vi "Extended Actor Template-Core_Process.vi"(0 "FTW Actor Instance Configuration":string="{\n  \"Identity\": \"ActorName\",\n  \"InboxAddress\": \"inproc://*\",\n  \"LoggerAddress\": \"\",\n  \"DebugEnableInboxLogging\": false,\n  \"DebugEnableJobLogging\": false,\n  \"LauncherAddress\": \"\",\n  \"Connections\": {\n    \"ConnectionOne\": \"inproc://connection-one\",\n    \"ConnectionTwo\": \"tcp://localhost/connection-two\"\n  },\n  \"Publishers\": {\n    \"PublisherOne\": \"inproc://publisher-one\",\n    \"PublisherTwo\": \"tcp://localhost/publisher-two\"\n  },\n  \"Subscriptions\": {\n    \"SubscriptionOne\": \"inproc://subscription-one\",\n    \"SubscriptionTwo\": \"tcp://localhost/subscription-two\"\n  },\n  \"My Data\": false,\n  \"Refresh Period\": 2\n}", 11 "ErrorIn":errorcluster) -> (15 "Error":errorcluster)   [LabVIEW 2013, in "Extended Actor Template-Core.lvclass"]
uses:
  Extended Actor Template-Core.lvclass
  source/actor/Message/Base/FTW-Message.lvclass
  Extended Actor Template-Core.lvclass/Extended Actor Template-Core.ctl
  source/actor/Instance/FTW-ActorInstance.lvclass/FTW-ActorInstance.ctl
  source/actor/JobSequencer/FTW-SEQ-Current.vi
  source/actor/Instance/FTW-ActorInstance.lvclass
  source/actor/Message/Request/FTW-Message-IncomingRequest.lvclass
  source/actor/Instance-Extended/FTW-ActorExtended.lvclass
panel:
  # "#TODO\nhide controls for a GUI"
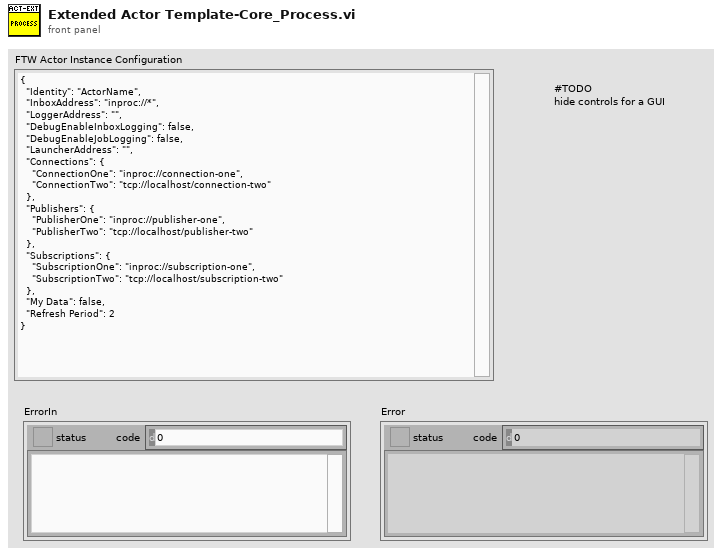
[diagram p1: front panel]
types:
  T1 = cluster{"Incoming Requests":refnum<event-registration>, "Local Messages":refnum<event-registration>, "Subscriber Registration":refnum<event-registration>}
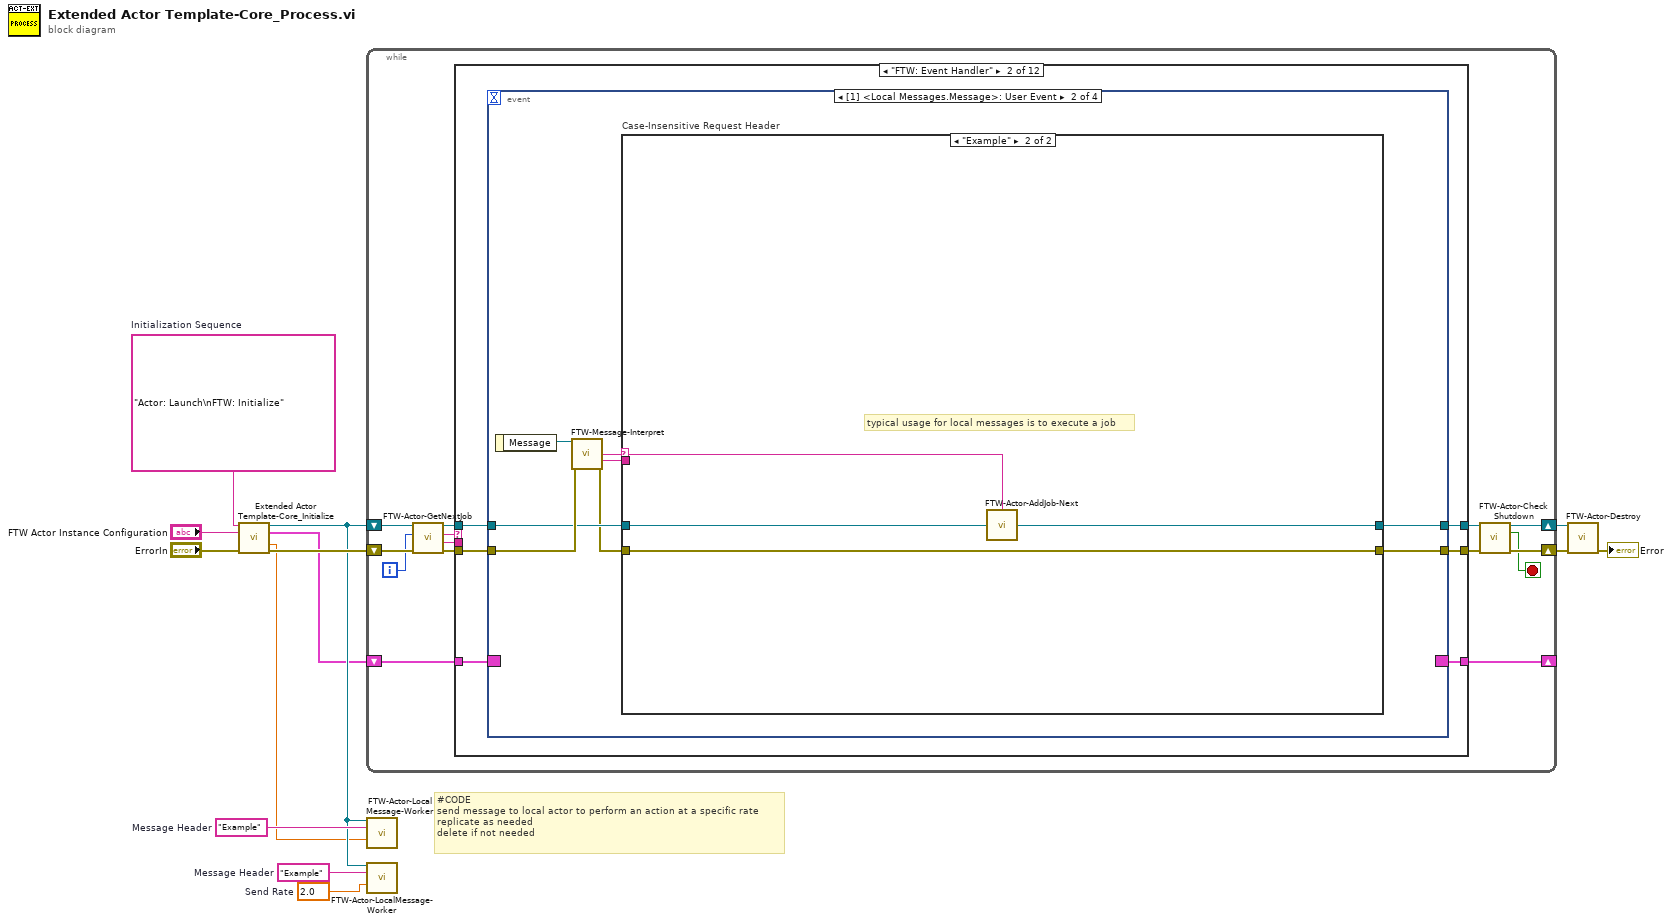
[diagram p0: block diagram]
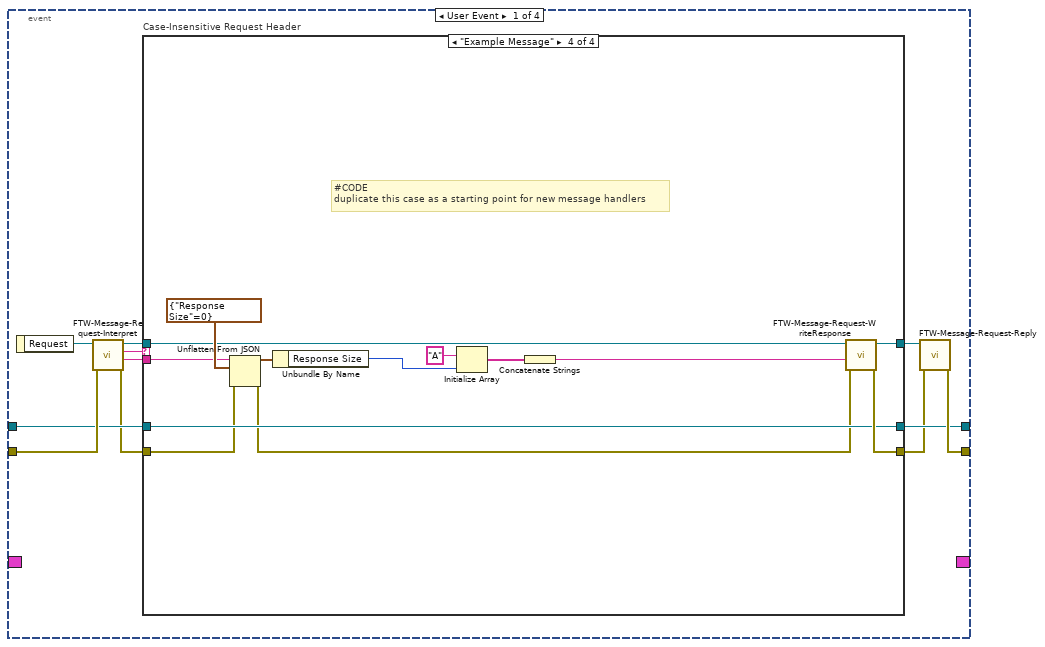
[diagram p3: hidden frame]
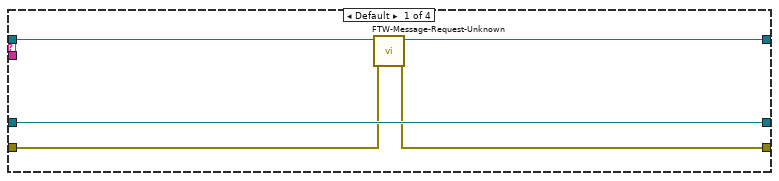
[diagram p4: hidden frame]
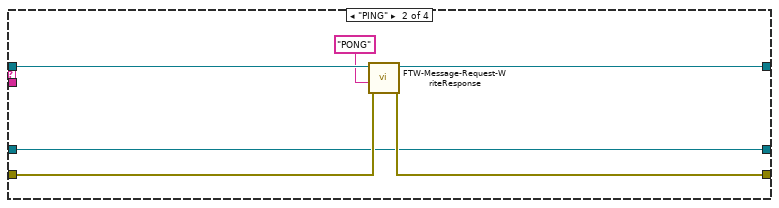
[diagram p5: hidden frame]
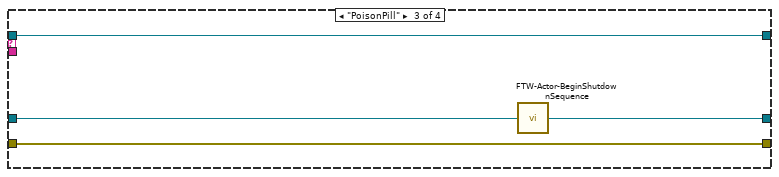
[diagram p6: hidden frame]
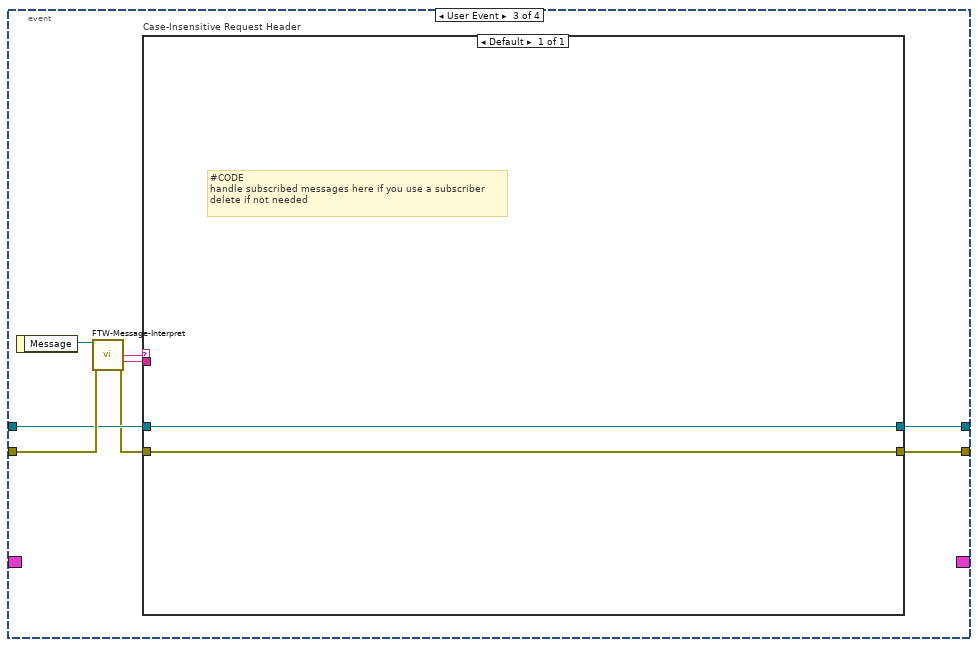
[diagram p8: hidden frame]
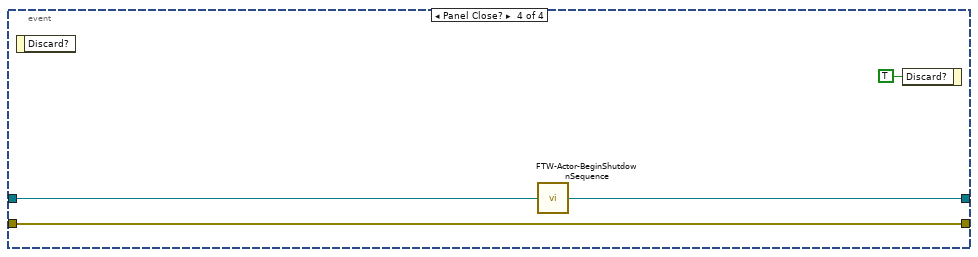
[diagram p9: hidden frame]
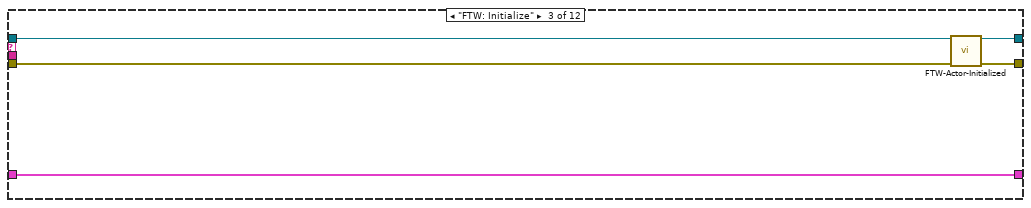
[diagram p10: hidden frame]
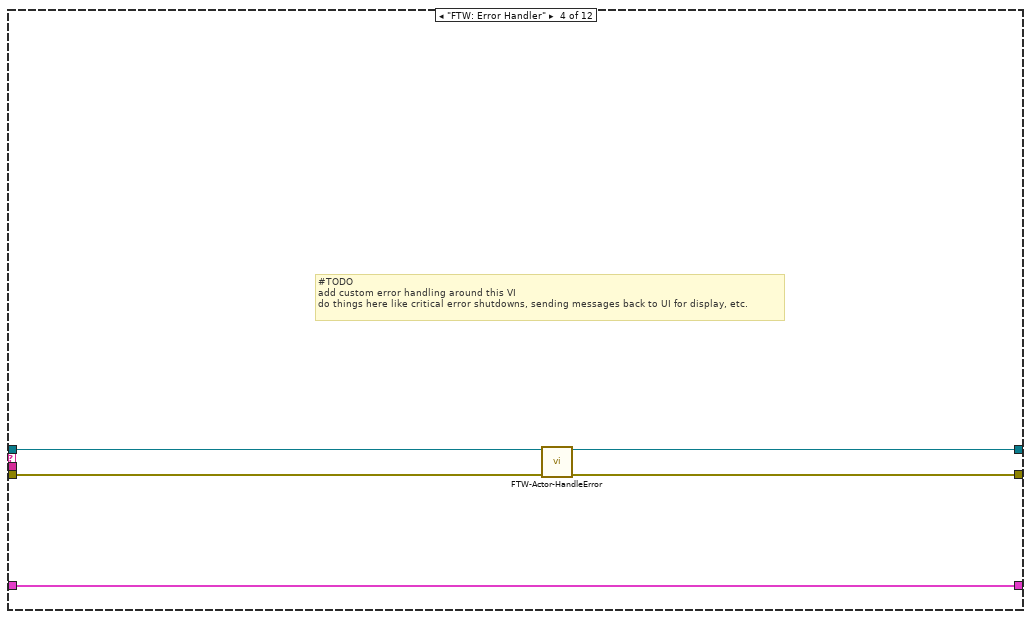
[diagram p11: hidden frame]
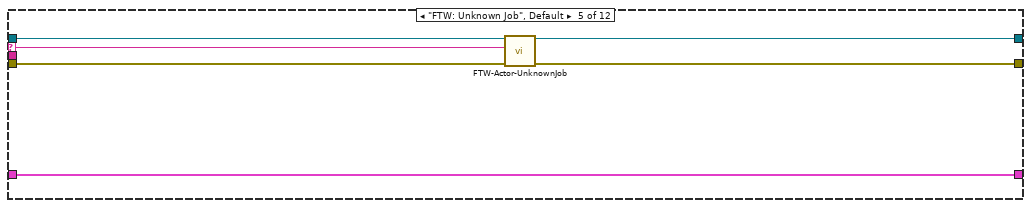
[diagram p12: hidden frame]
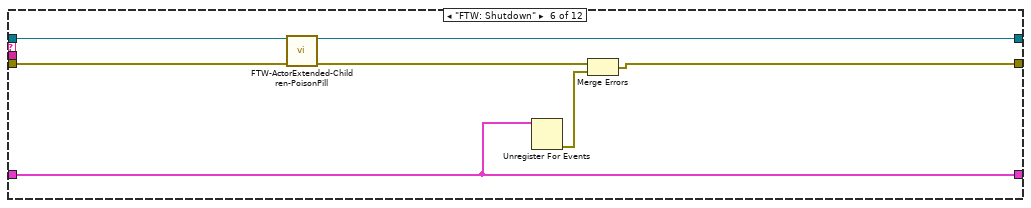
[diagram p13: hidden frame]
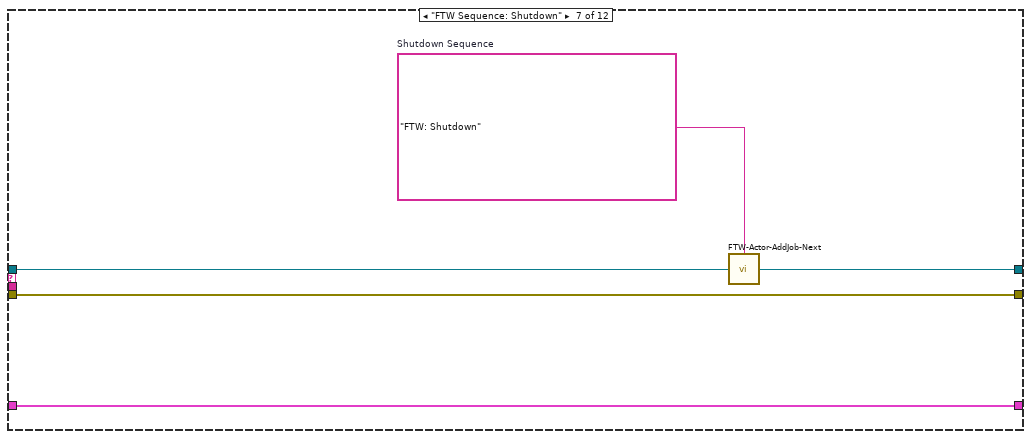
[diagram p14: hidden frame]
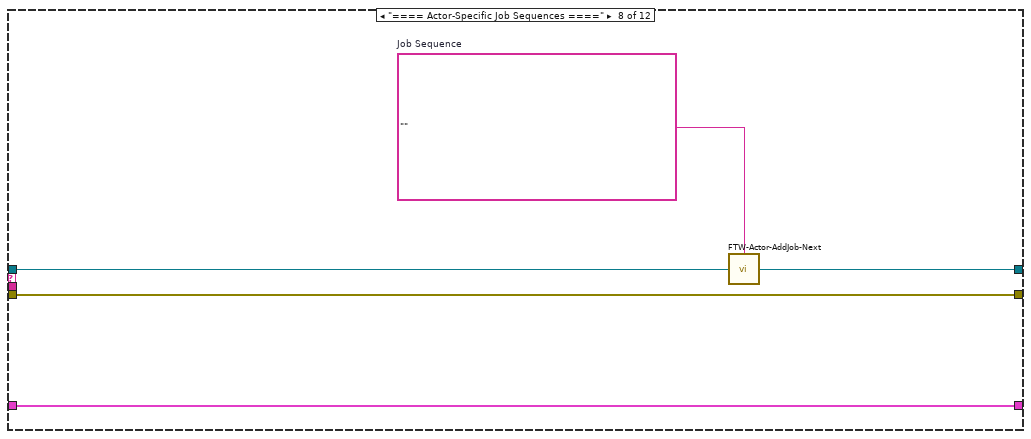
[diagram p15: hidden frame]
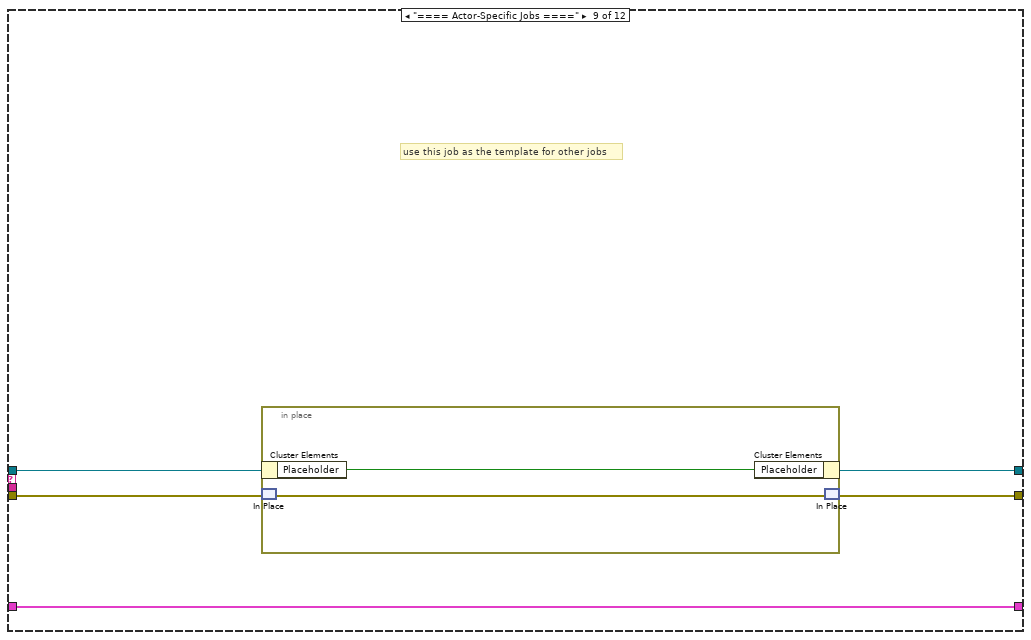
[diagram p16: hidden frame]
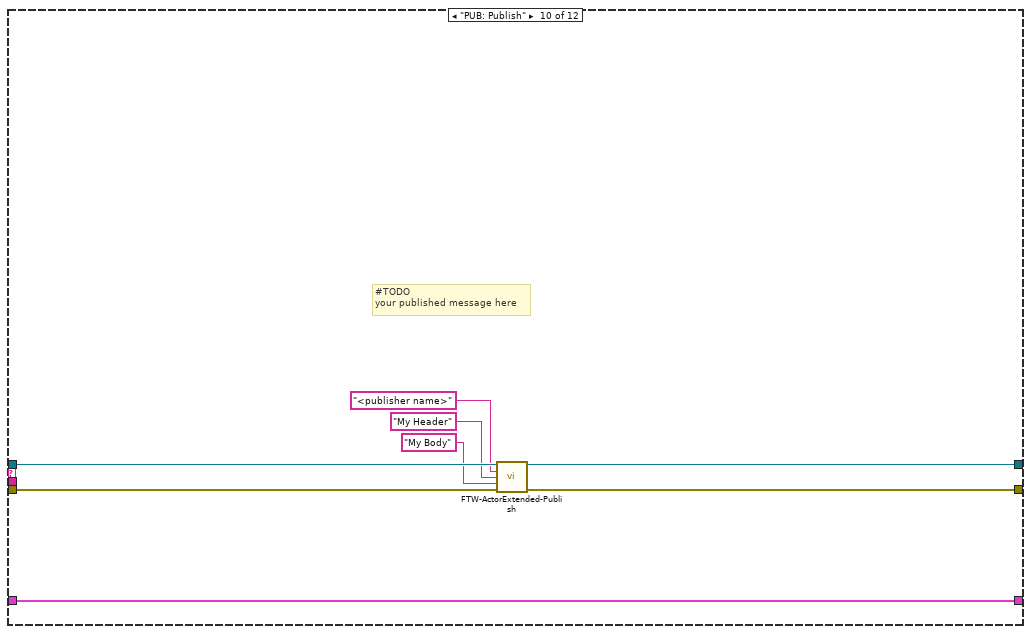
[diagram p17: hidden frame]
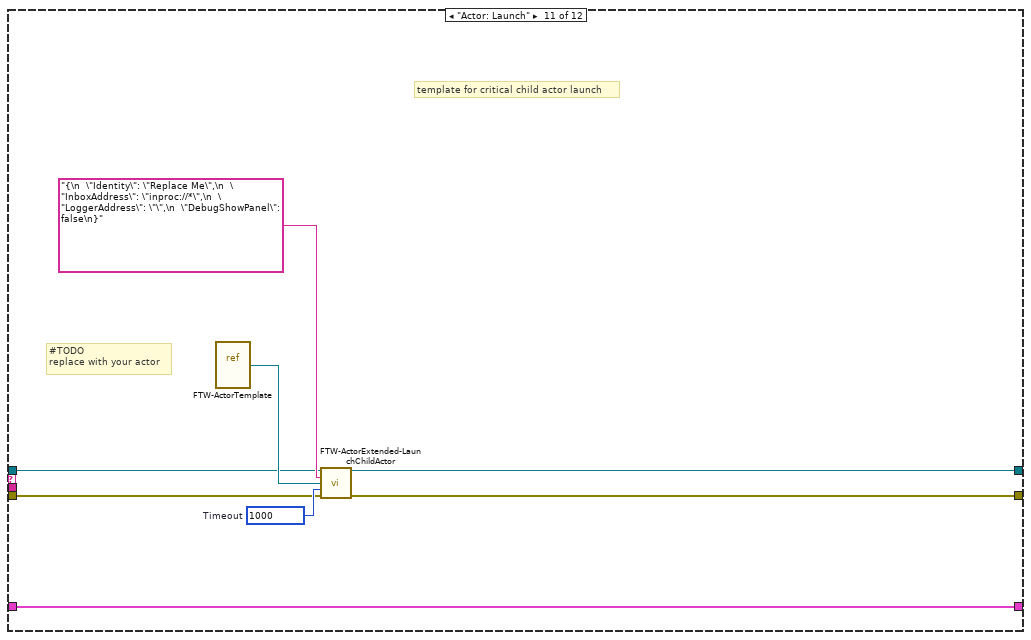
[diagram p18: hidden frame]
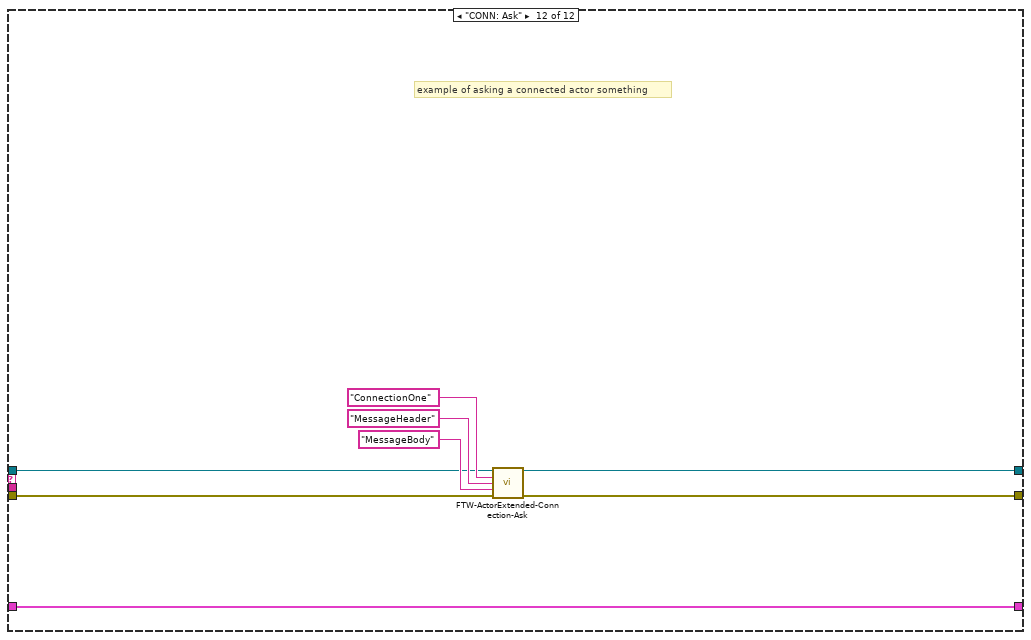
[diagram p19: hidden frame]
diagram:
  w5 = 2.0  # Send Rate
  w4 = "Example"  # Message Header
  w6 = "Example"  # Message Header
  w9 = "Actor: Launch\nFTW: Initialize"  # Initialization Sequence
  # "#CODE\nsend message to local actor to perform an action at a specific rate\nreplicate as needed\ndelete if not needed"
  n1 = call "Extended Actor Template-Core_Initialize.vi"("Initialization Sequence"=w9, "FTW Actor Instance Configuration"="FTW Actor Instance Configuration", "error in (no error)"="ErrorIn") -> ("Actor Template-Core out"=w3:refnum<class "Extended Actor Template-Core.lvclass">, "Event Refnums"=w1:T1, "Refresh Period"=w2:dbl, "error out"=w10:errorcluster)  [unwired: 9 in]
  n2 = while {
    shift-right: [w17] -> w12
    shift-left: w10 -> [w24]
    shift-right: [w14] -> _
    shift-left: w1 -> [w27]
    shift-right: [w19] -> w13
    shift-left: w3 -> [w26]
    i -> [w15]
    stop <- w16 stop-if-true
    n3 = call "FTW-Actor-GetNextJob.vi"("error in"=w24, "Jobs Performed"=w15, "FTW Actor Instance"=w26) -> ("error out"=w23:errorcluster, "Job Data"=w21:string, "Job Name"=w22:string, "FTW Actor Instance out"=w25:refnum<class "Extended Actor Template-Core.lvclass">)  [unwired: 5 in]
    n4 = case shown="\"FTW: Event Handler\"" w22 {
      selector: w22 -> [_ _ _ _ w114 _ _ _ _ _ _ _]
      tunnel: [w29 w36 w105 w109 w117 w125 w130 w135 w139 w149 w154 w160] -> w18
      tunnel: w23 -> [w29 w35 w107 w111 w118 w126 w130 w135 w140 w150 w155 w163]
      tunnel: w27 -> [w30 w31 w108 w113 w119 w123 w131 w136 w141 w151 w159 w167]
      tunnel: [w30 w34 w108 w113 w119 w123 w131 w136 w141 w151 w159 w167] -> w14
      tunnel: w21 -> [_ _ _ _ _ _ _ _ _ _ _ _]
      tunnel: [w28 w33 w106 w110 w115 w120 w128 w133 w137 w147 w152 w161] -> w20
      tunnel: w25 -> [w28 w32 w104 w112 w116 w121 w129 w134 w138 w148 w153 w162]
      frame "==== Featherweight Framework Jobs ====" {
      }
      frame "FTW: Event Handler" {
        n5 = event shown="[1] <Local Messages.Message>: User Event" {
          selector: w31 -> [_ _ _ _]
          dyn-events: [_ _ _ _] -> w34
          timeout: _ -> [_ _ _ _]
          tunnel: [w46 w78 w92 w102] -> w36
          tunnel: w35 -> [w45 w82 w96 w102]
          tunnel: [w40 w79 w93 w100] -> w33
          tunnel: w32 -> [w44 w81 w95 w101]
          event User Event {
            n6 = event-data() -> ("Request"=w47:refnum<class "FTW-Message-IncomingRequest.lvclass">)  [unwired: 1 in]
            n7 = call "FTW-Message-Request-Interpret.vi"("error in"=w45, "FTW Incoming Request"=w47) -> ("error out"=w43:errorcluster, "Request Body"=w37:string, "Request Header"=w41:string, "FTW Incoming Request out"=w42:refnum<class "FTW-Message-IncomingRequest.lvclass">)  [unwired: 6 in]
            n8 = case "Case-Insensitive Request Header" shown="\"Example Message\"" w41 {
              tunnel: [w50 w56 w61 w75] -> w39
              tunnel: w43 -> [w51 w57 w61 w64]
              tunnel: [w52 w55 w62 w73] -> w40
              tunnel: w44 -> [w52 w55 w60 w73]
              tunnel: w42 -> [w49 w58 w59 w65]
              tunnel: [w48 w54 w59 w74] -> w38
              tunnel: w37 -> [_ _ _ w63]
              frame Default {
                n9 = call "FTW-Message-Request-Unknown.vi"("error in"=w51, "FTW Incoming Request"=w49) -> ("error out"=w50:errorcluster, "FTW Incoming Request Out"=w48:refnum<class "FTW-Message-IncomingRequest.lvclass">)  [unwired: 8 in]
              }
              frame "PING" {
                n10 = call "FTW-Message-Request-WriteResponse.vi"("error in"=w57, "Response Body"="PONG" ("Response Header"), "FTW Incoming Request"=w58) -> ("error out"=w56:errorcluster, "FTW Incoming Request out"=w54:refnum<class "FTW-Message-IncomingRequest.lvclass">)  [unwired: 7 in]
              }
              frame "PoisonPill" {
                n11 = call "FTW-Actor-BeginShutdownSequence.vi"("FTW Actor Instance"=w60) -> ("FTW Actor Instance out"=w62:refnum<class "Extended Actor Template-Core.lvclass">)  [unwired: 3 in]
              }
              frame "Example Message" {
                # "#CODE\nduplicate this case as a starting point for new message handlers"
                n12 = Unflatten From JSON(JSON string=w63, type and defaults=cluster{"Response Size":i32} {"Response Size"=0}, error in (no error)=w64) -> (value=w70:cluster{"Response Size":i32}, error out=w72:errorcluster)  [unwired: 4 in]
                n13 = Unbundle By Name(w70) -> ("Response Size"=w69:i32)
                n14 = Initialize Array("A", w69) -> (w67:string[])
                n15 = Concatenate Strings(w67) -> (w66:string)
                n16 = call "FTW-Message-Request-WriteResponse.vi"("error in"=w72, "Response Body"=w66, "FTW Incoming Request"=w65) -> ("error out"=w75:errorcluster, "FTW Incoming Request out"=w74:refnum<class "FTW-Message-IncomingRequest.lvclass">)  [unwired: 7 in]
              }
            }
            n17 = call "FTW-Message-Request-Reply.vi"("FTW: Reply Error"=w39, "FTW Incoming Request"=w38) -> ("error out"=w46:errorcluster)  [unwired: 8 in, 1 out]
          }
          event User Event {
            n18 = event-data() -> ("Message"=w83:refnum<class "FTW-Message.lvclass">)  [unwired: 1 in]
            n19 = call-dynamic "FTW-Message-Interpret.vi"("FTW Message"=w83, "error in"=w82) -> ("Message Header"=w77:string, "Message Body"=w76:string, "error out"=w80:errorcluster)  [unwired: 9 in, 2 out]
            n20 = case "Case-Insensitive Request Header" shown="\"Example\"" w77 {
              selector: w77 -> [_ w86]
              tunnel: [w84 w88] -> w78
              tunnel: w80 -> [w84 w88]
              tunnel: [w85 w87] -> w79
              tunnel: w81 -> [w85 w89]
              tunnel: w76 -> [_ _]
              frame Default {
                # "#CODE\nhandle local messages here\ndelete if not needed"
              }
              frame "Example" {
                # "typical usage for local messages is to execute a job"
                n21 = call "FTW-Actor-AddJob-Next.vi"("Add Next in Job Queue"=w86, "FTW Actor Instance"=w89) -> ("FTW Actor Instance out"=w87:refnum<class "Extended Actor Template-Core.lvclass">)  [unwired: 2 in]
              }
            }
          }
          event User Event {
            n22 = event-data() -> ("Message"=w97:refnum<class "FTW-Message.lvclass">)  [unwired: 1 in]
            n23 = call-dynamic "FTW-Message-Interpret.vi"("FTW Message"=w97, "error in"=w96) -> ("Message Header"=w91:string, "Message Body"=w90:string, "error out"=w94:errorcluster)  [unwired: 9 in, 2 out]
            n24 = case "Case-Insensitive Request Header" shown="Default" w91 {
              tunnel: [w98] -> w92
              tunnel: w94 -> [w98]
              tunnel: [w99] -> w93
              tunnel: w95 -> [w99]
              tunnel: w90 -> [_]
              frame Default {
                # "#CODE\nhandle subscribed messages here if you use a subscriber\ndelete if not needed"
              }
            }
          }
          event Panel Close? {
            n25 = event-data() -> ()  [unwired: 1 in, 1 out]
            n26 = call "FTW-Actor-BeginShutdownSequence.vi"("FTW Actor Instance"=w101) -> ("FTW Actor Instance out"=w100:refnum<class "Extended Actor Template-Core.lvclass">)  [unwired: 3 in]
            n27 = event-data("Discard?"=TRUE) -> ()  [unwired: 1 in, 1 out]
          }
        }
      }
      frame "FTW: Initialize" {
        n28 = call-dynamic "FTW-Actor-Initialized.vi"("FTW Actor Instance"=w104, "error in"=w107) -> ("FTW Actor Instance out"=w106:refnum<class "Extended Actor Template-Core.lvclass">, "error out"=w105:errorcluster)  [unwired: 12 in]
      }
      frame "FTW: Error Handler" {
        # "#TODO\nadd custom error handling around this VI\ndo things here like critical error shutdowns, sending messages back to UI for display, etc."
        n29 = call-dynamic "FTW-Actor-HandleError.vi"("FTW Actor Instance"=w112, "error in"=w111) -> ("FTW Actor Instance out"=w110:refnum<class "Extended Actor Template-Core.lvclass">, "error out"=w109:errorcluster)  [unwired: 10 in, 2 out]
      }
      frame "FTW: Unknown Job", Default {
        n30 = call-dynamic "FTW-Actor-UnknownJob.vi"("FTW Actor Instance"=w116, "Unknown Job"=w114, "error in"=w118) -> ("FTW Actor Instance out"=w115:refnum<class "Extended Actor Template-Core.lvclass">, "error out"=w117:errorcluster)  [unwired: 11 in]
      }
      frame "FTW: Shutdown" {
        n31 = call "FTW-ActorExtended-Children-PoisonPill.vi"("FTW-ActorExtended In"=w121, "error in"=w126) -> ("FTW-ActorExtended Out"=w120:refnum<class "Extended Actor Template-Core.lvclass">, "error out"=w122:errorcluster)  [unwired: 12 in]
        n32 = Unregister For Events(event registration refnum=w123) -> (error out=w124:errorcluster)  [unwired: 1 in]
        n33 = Merge Errors(w122, w124) -> (w125:errorcluster)
      }
      frame "FTW Sequence: Shutdown" {
        w127 = "FTW: Shutdown"  # Shutdown Sequence
        n34 = call "FTW-Actor-AddJob-Next.vi"("Add Next in Job Queue"=w127, "FTW Actor Instance"=w129) -> ("FTW Actor Instance out"=w128:refnum<class "Extended Actor Template-Core.lvclass">)  [unwired: 2 in]
      }
      frame "==== Actor-Specific Job Sequences ====" {
        w132 = ""  # Job Sequence
        n35 = call "FTW-Actor-AddJob-Next.vi"("Add Next in Job Queue"=w132, "FTW Actor Instance"=w134) -> ("FTW Actor Instance out"=w133:refnum<class "Extended Actor Template-Core.lvclass">)  [unwired: 2 in]
      }
      frame "==== Actor-Specific Jobs ====" {
        # "use this job as the template for other jobs"
        n36 = in-place {
          n37 = in-place-cluster #1(w138) -> ("Placeholder"=w142:bool)
          n38 = in-place-match #2(w140) -> (w143:errorcluster)
          n39 = in-place-cluster #1("Placeholder"=w142) -> (w137:refnum<class "Extended Actor Template-Core.lvclass">)
          n40 = in-place-match #2(w143) -> (w139:errorcluster)
        }
      }
      frame "PUB: Publish" {
        # "#TODO\nyour published message here"
        n41 = call "FTW-ActorExtended-Publish.vi"("FTW-ActorExtended In"=w148, "Publisher Name"="<publisher name>", "Message Header"="My Header" ("Header"), "Message Body"="My Body" ("Header"), "error in"=w150) -> ("FTW-ActorExtended Out"=w147:refnum<class "Extended Actor Template-Core.lvclass">, "error out"=w149:errorcluster)  [unwired: 9 in]
      }
      frame "Actor: Launch" {
        w158 = 1000  # Timeout
        # "#TODO\nreplace with your actor"
        # "template for critical child actor launch"
        n42 = vi-ref "FTW-ActorTemplate.vi"() -> (w157:refnum<vi>)
        n43 = call "FTW-ActorExtended-LaunchChildActor.vi"("FTW Actor Connector Type"=w153, "Configuration"="{\n  \"Identity\": \"Replace Me\",\n  \"InboxAddress\": \"inproc://*\",\n  \"LoggerAddress\": \"\",\n  \"DebugShowPanel\": false\n}", "Actor VI Refnum"=w157, "Timeout"=w158, "error in"=w155) -> ("FTW-ActorExtended.lvclass"=w152:refnum<class "Extended Actor Template-Core.lvclass">, "error out"=w154:errorcluster)  [unwired: 7 in, 2 out]
      }
      frame "CONN: Ask" {
        # "example of asking a connected actor something"
        n44 = call "FTW-ActorExtended-Connection-Ask.vi"("FTW-ActorExtended In"=w162, "Connector Name"="ConnectionOne" ("Publisher Name"), "Message Header"="MessageHeader", "Message Body"="MessageBody", "error in"=w163) -> ("FTW-ActorExtended Out"=w161:refnum<class "Extended Actor Template-Core.lvclass">, "error out"=w160:errorcluster)  [unwired: 5 in, 4 out]
      }
    }
    n45 = call "FTW-Actor-CheckShutdown.vi"("FTW Actor Instance"=w20, "error in"=w18) -> ("FTW Actor Instance out"=w19:refnum<class "Extended Actor Template-Core.lvclass">, "Shutdown?"=w16:bool, "error out"=w17:errorcluster)  [unwired: 11 in]
  }
  n46 = call-dynamic "FTW-Actor-LocalMessage-Worker.vi"("FTW-ActorInstance In"=w3, "Message Header"=w6, "Send Rate"=w2) -> ()  [unwired: 13 in]
  n47 = call-dynamic "FTW-Actor-LocalMessage-Worker.vi"("FTW-ActorInstance In"=w3, "Message Header"=w4, "Send Rate"=w5) -> ()  [unwired: 13 in]
  n48 = call-dynamic "FTW-Actor-Destroy.vi"("FTW Actor Instance"=w13, "error in"=w12) -> ("error out"=→"Error":errorcluster)  [unwired: 13 in]
